vi "PM-A-myDAQ-close.vi"(8 "error in (no error)":errorcluster, 11 "Refnum in":refnum<k21>) -> (0 "error out":errorcluster)   [LabVIEW 2020]
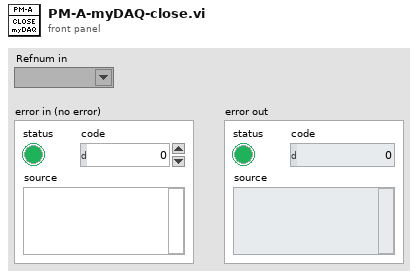
[diagram p1: front panel]
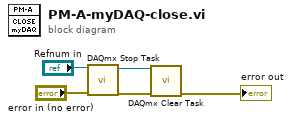
[diagram p0: block diagram]
diagram:
  n1 = call <vilib>:"DAQmx Stop Task.vi"("task/channels in"="Refnum in", "error in"="error in (no error)") -> ("task out"=w2:refnum<k21>, "error out"=w3:errorcluster)  [unwired: 12 in]
  n2 = call <vilib>:"DAQmx Clear Task.vi"("task in"=w2, "error in"=w3) -> ("error out"=→"error out":errorcluster)  [unwired: 13 in]
